vi "convert.vi"(8 "error in (no error)":errorcluster, 10 "Input":dbl, 11 "ConvertDACRawToEngStrategy in":refnum<class "ConvertDACRawToEngStrategy.lvclass">) -> (0 "error out":errorcluster, 2 "Output":dbl, 3 "ConvertDACRawToEngStrategy out":refnum<class "ConvertDACRawToEngStrategy.lvclass">)   [LabVIEW 2015, in "ConvertDACRawToEngStrategy.lvclass"]
uses:
  ConvertDACRawToEngStrategy.lvclass
  ConvertDACRawToEngStrategy.lvclass/ConvertDACRawToEngStrategy.ctl
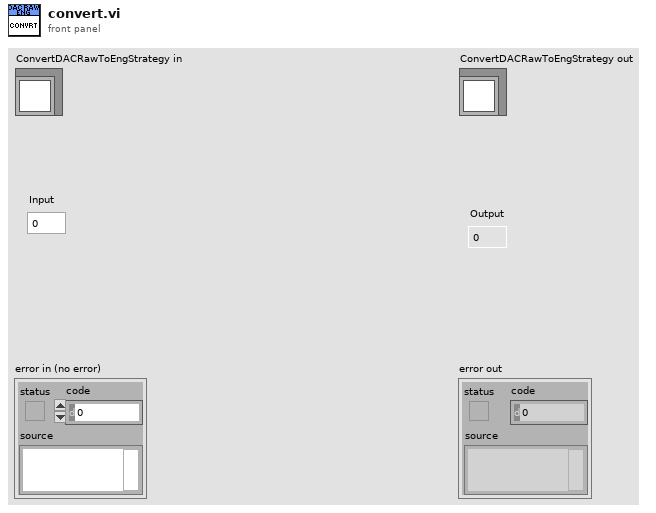
[diagram p1: front panel]
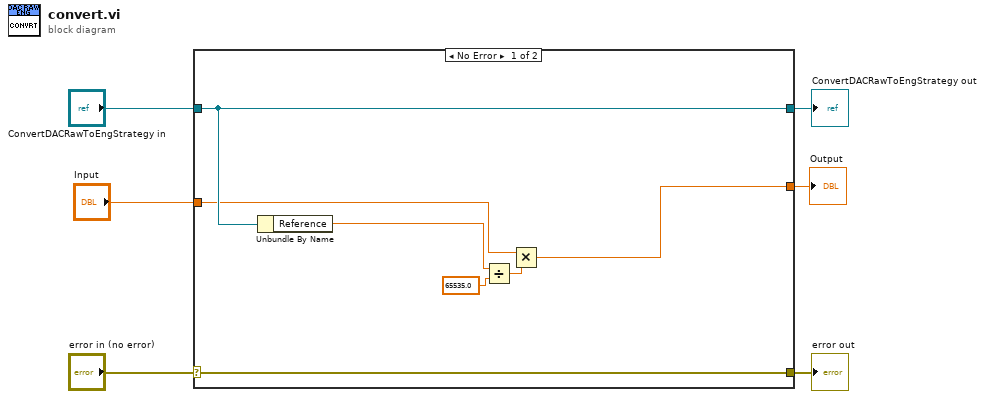
[diagram p0: block diagram]
diagram:
  n1 = case shown="No Error" "error in (no error)" {
    selector: "error in (no error)" -> [w8 w16]
    tunnel: [w8 w16] -> w5
    tunnel: [w11 w15] -> w3
    tunnel: "ConvertDACRawToEngStrategy in" -> [w11 w15]
    tunnel: "Input" -> [w10 w14]
    tunnel: [w9 w14] -> w1
    frame No Error {
      n2 = Unbundle By Name(w11) -> ("Reference"=w7:dbl)
      n3 = Divide(x=w7, y=65535.0) -> (x/y=w13:dbl)
      n4 = Multiply(x=w10, y=w13) -> (x*y=w9:dbl)
    }
    frame Error {
    }
  }
  "error out" <- w5
  "ConvertDACRawToEngStrategy out" <- w3
  "Output" <- w1
